vi "Topo & GridSpectr_DriftCorrection_v5.1- Cloud.vi"(6 "Internal use":string, 7 "Grid param":T2 {"height (m)" format="%#_6p"; "width (m)" format="%#_6p"; "center Y (m)" format="%#_6p"; "center X (m)" format="%#_6p"}, 8 "Error in (no error)":errorcluster, 9 "Points Y/Index Y":i32, 10 "Points X/Index X":i32, 11 "Method":enum16{"init", "run", "end"}(ring)=enum."end") -> (0 "Error out":errorcluster)   [LabVIEW 2014]
doc: "Example of a measurement VI to be used in the \"Experiments on a Grid\" tool as external VI.\n\nThis example measure the topography and spectroscopy data. The spectroscopy measurements are taken on a subgrid. The data are saved to a sxm and a binary file.\n\n- Nanonis Programming Interface -"
uses:
  <userlib>/Nanonis Prog Interface V5/Nanonis Prog Interface.lvlib
panel:
  in  "Drift Correction":bool
  in  "Set Session":bool
  in  "STS current step":dbl format="%#_6p"
  in  "tip Speed (m/s)":sgl=1e-08 format="%.2p"
  in  "Drift Correction 2":T1
  out "X drift":i32
  out "Y drift":i32
  in  "Channel index (0-23)":u8=14
  in  "File name":string="_3_mol_Chain_single_mol_KONDO"
  in  "STS Current":dbl=2e-10 format="%#_6p"
  in  "Imaging Current":dbl=8e-11 format="%#_6p"
  in  "zdrift \nDuration (s)":dbl
  in  "Correct z drift":bool
  out "Status":string="init"
  in  "Drift correction Pixels":i32=256 caption="Pixels for drift correction"
  out "Y Offset":dbl
  out "X Offset":dbl
  out "Points taken":dbl
  in  "Drift Correction every":i32=10
  in  "Y subgrid spacing":u16=1
  in  "X subgrid spacing":u16=1
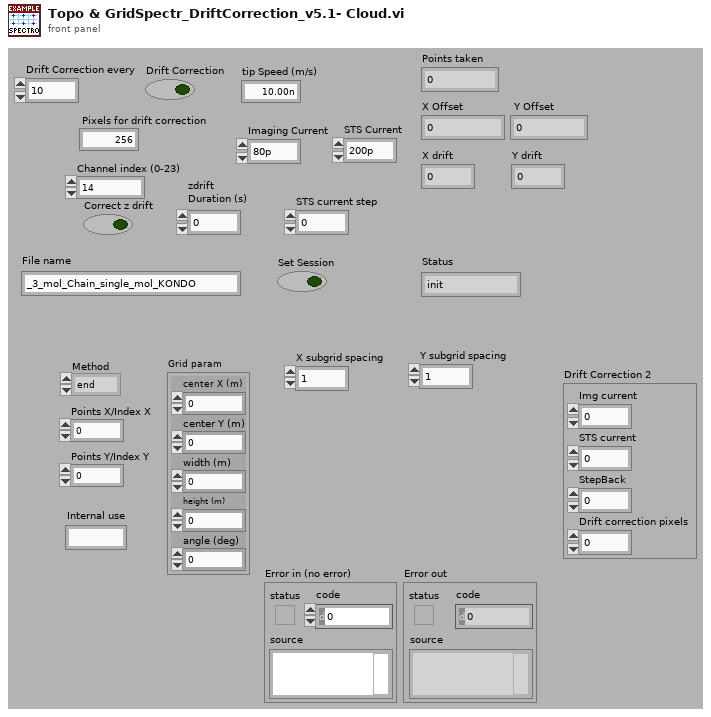
[diagram p1: front panel]
types:
  T1 = cluster{"Img current":dbl, "STS current":dbl, "StepBack":dbl, "Drift correction pixels":dbl}
  T2 = cluster{"center X (m)":sgl, "center Y (m)":sgl, "width (m)":sgl, "height (m)":sgl, "angle (deg)":sgl}
  T3 = enum16{"Header", "TOPO", "STS", "GRID", "GRIDCloud"}
  T4 = cluster{"center X":sgl, "center Y":sgl, "angle":sgl, "width":sgl, "height":sgl, "# pixels":i32, "# lines":i32}
  T5 = cluster{"Name":string, "Calibration":sgl, "Offset":sgl, "Channel index":i32}[]
  T6 = cluster{"up/down":bool, "time/line":sgl, "start time":timestamp, "end time":timestamp}
  T7 = cluster{"Z averaging time (s)":sgl, "Z offset (m)":sgl, "Initial settling time (s)":sgl}
  T8 = cluster{"Max. slew rate (V/s)":sgl, "Settling time (s)":sgl, "Integration time (s)":sgl}
  T9 = cluster{"End settling time (s)":sgl, "Z control time (s)":sgl}
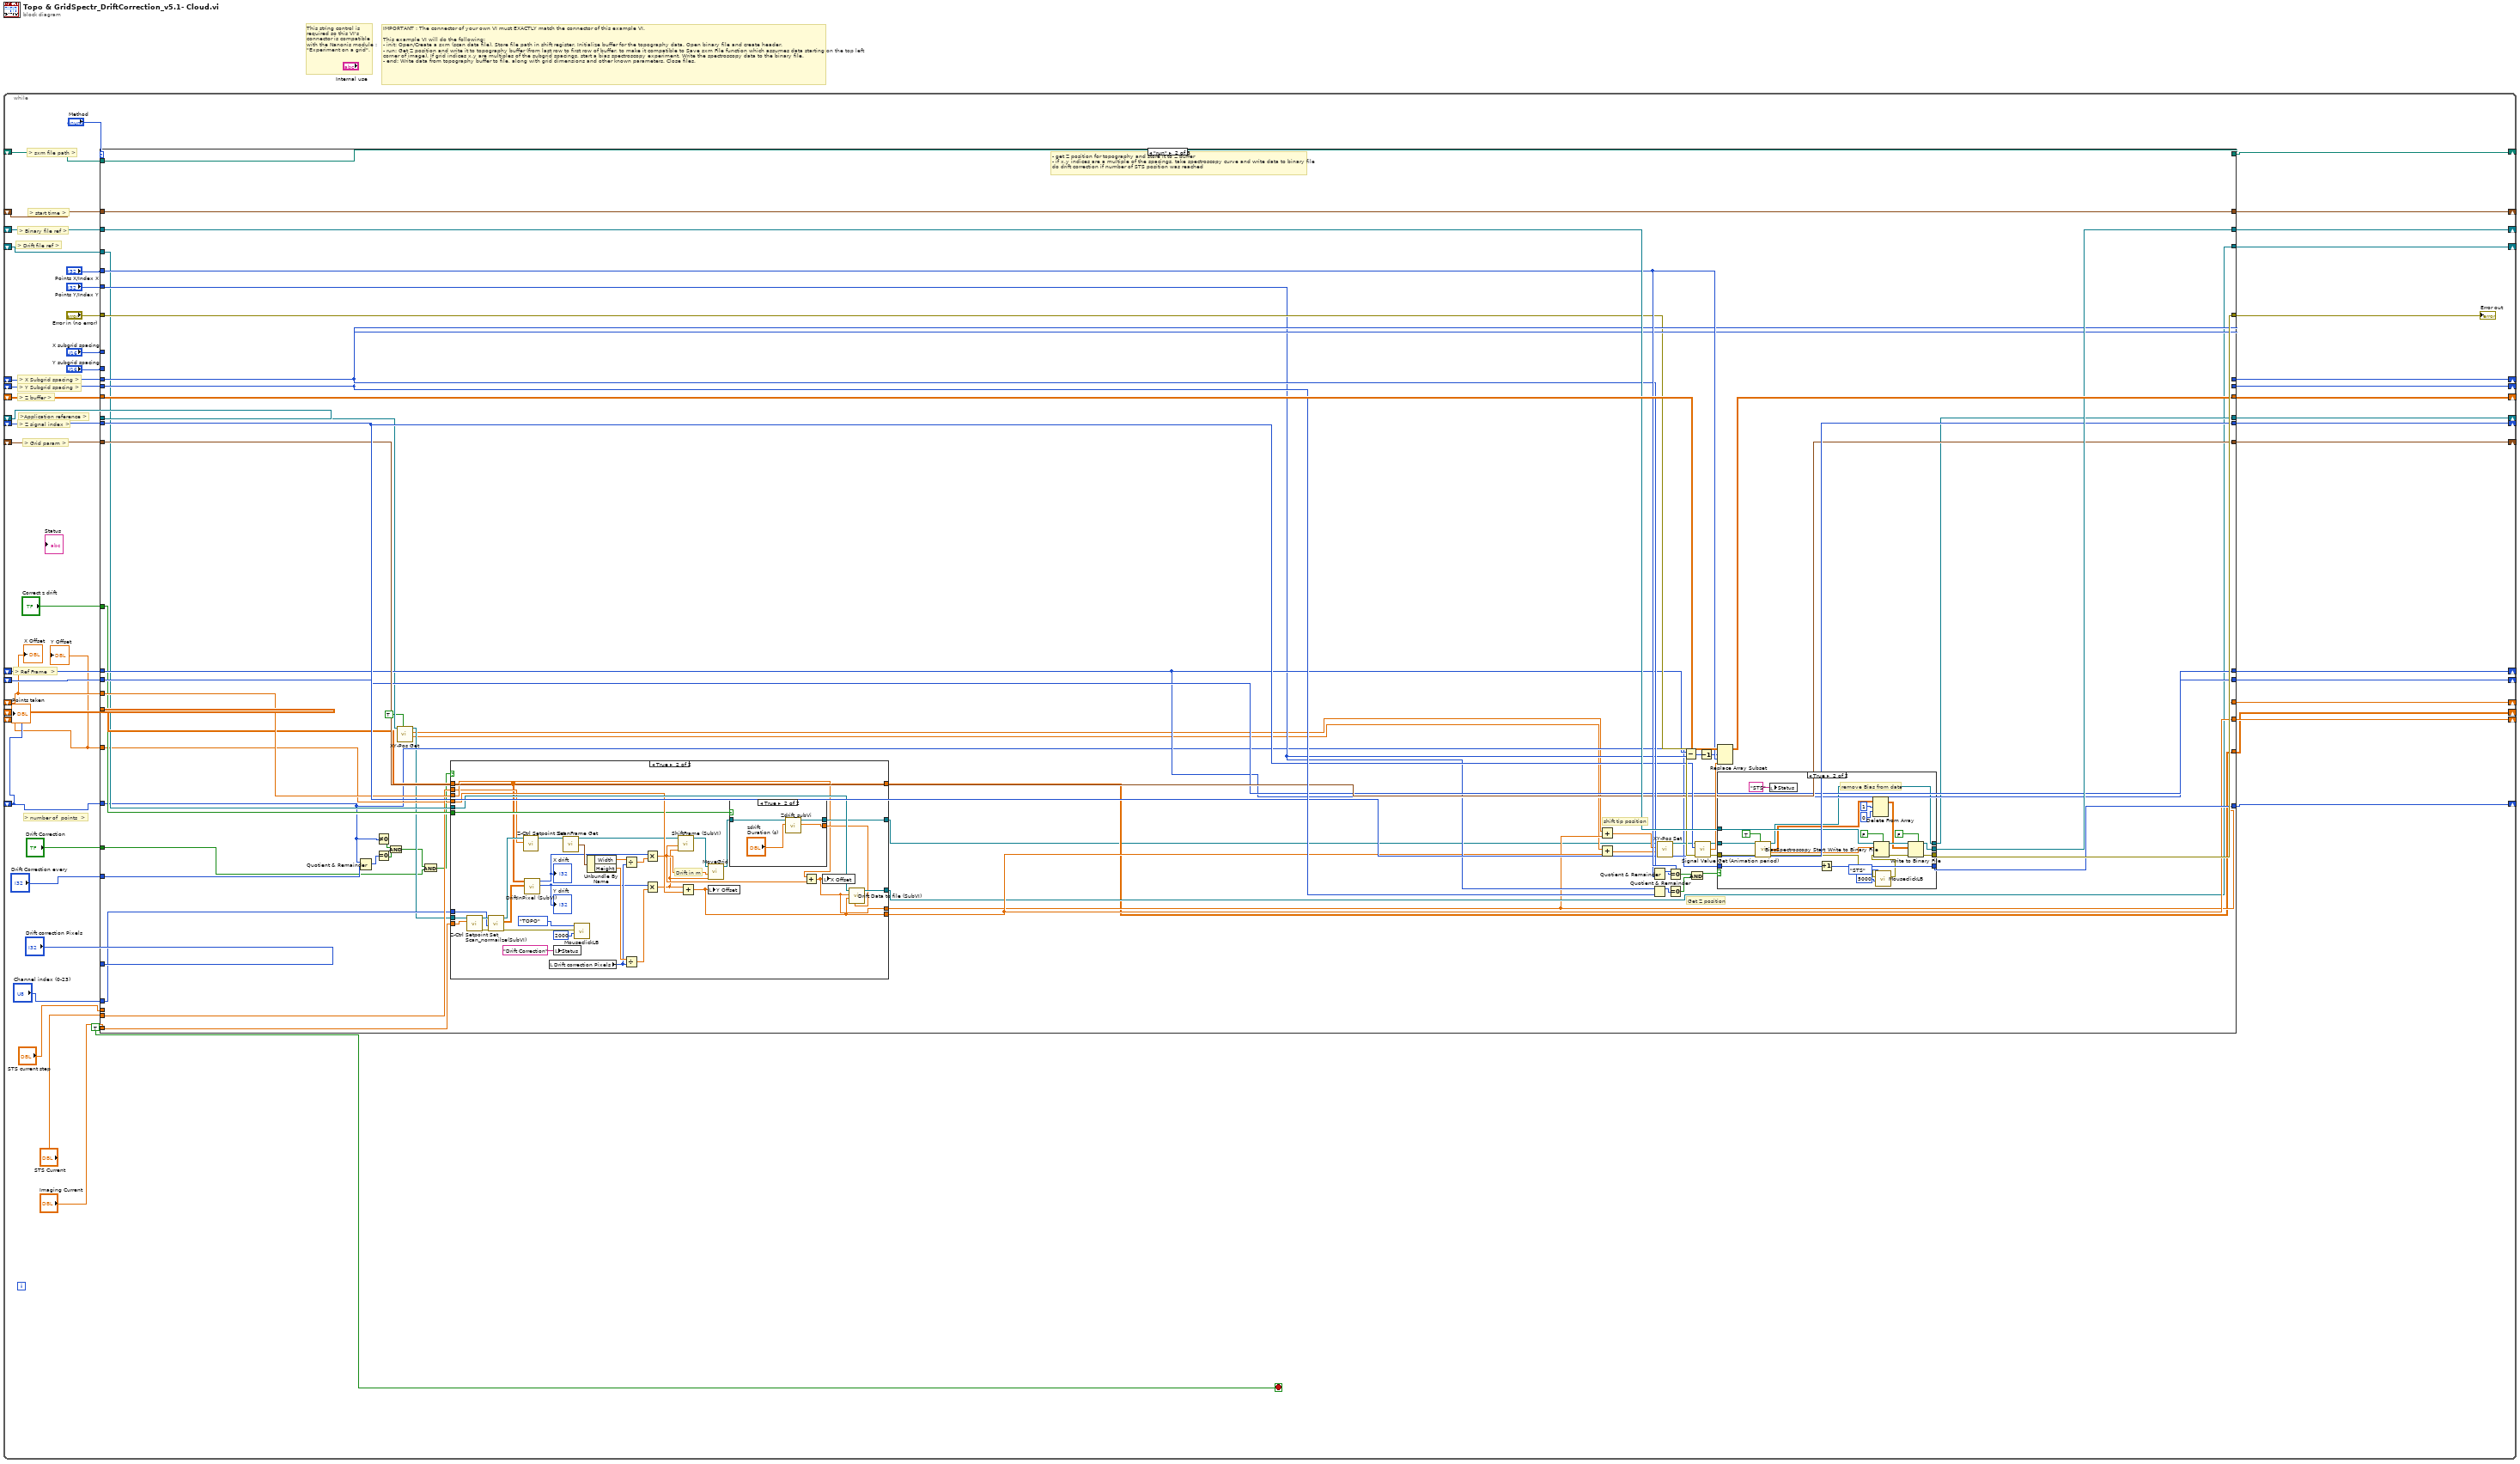
[diagram p0: block diagram]
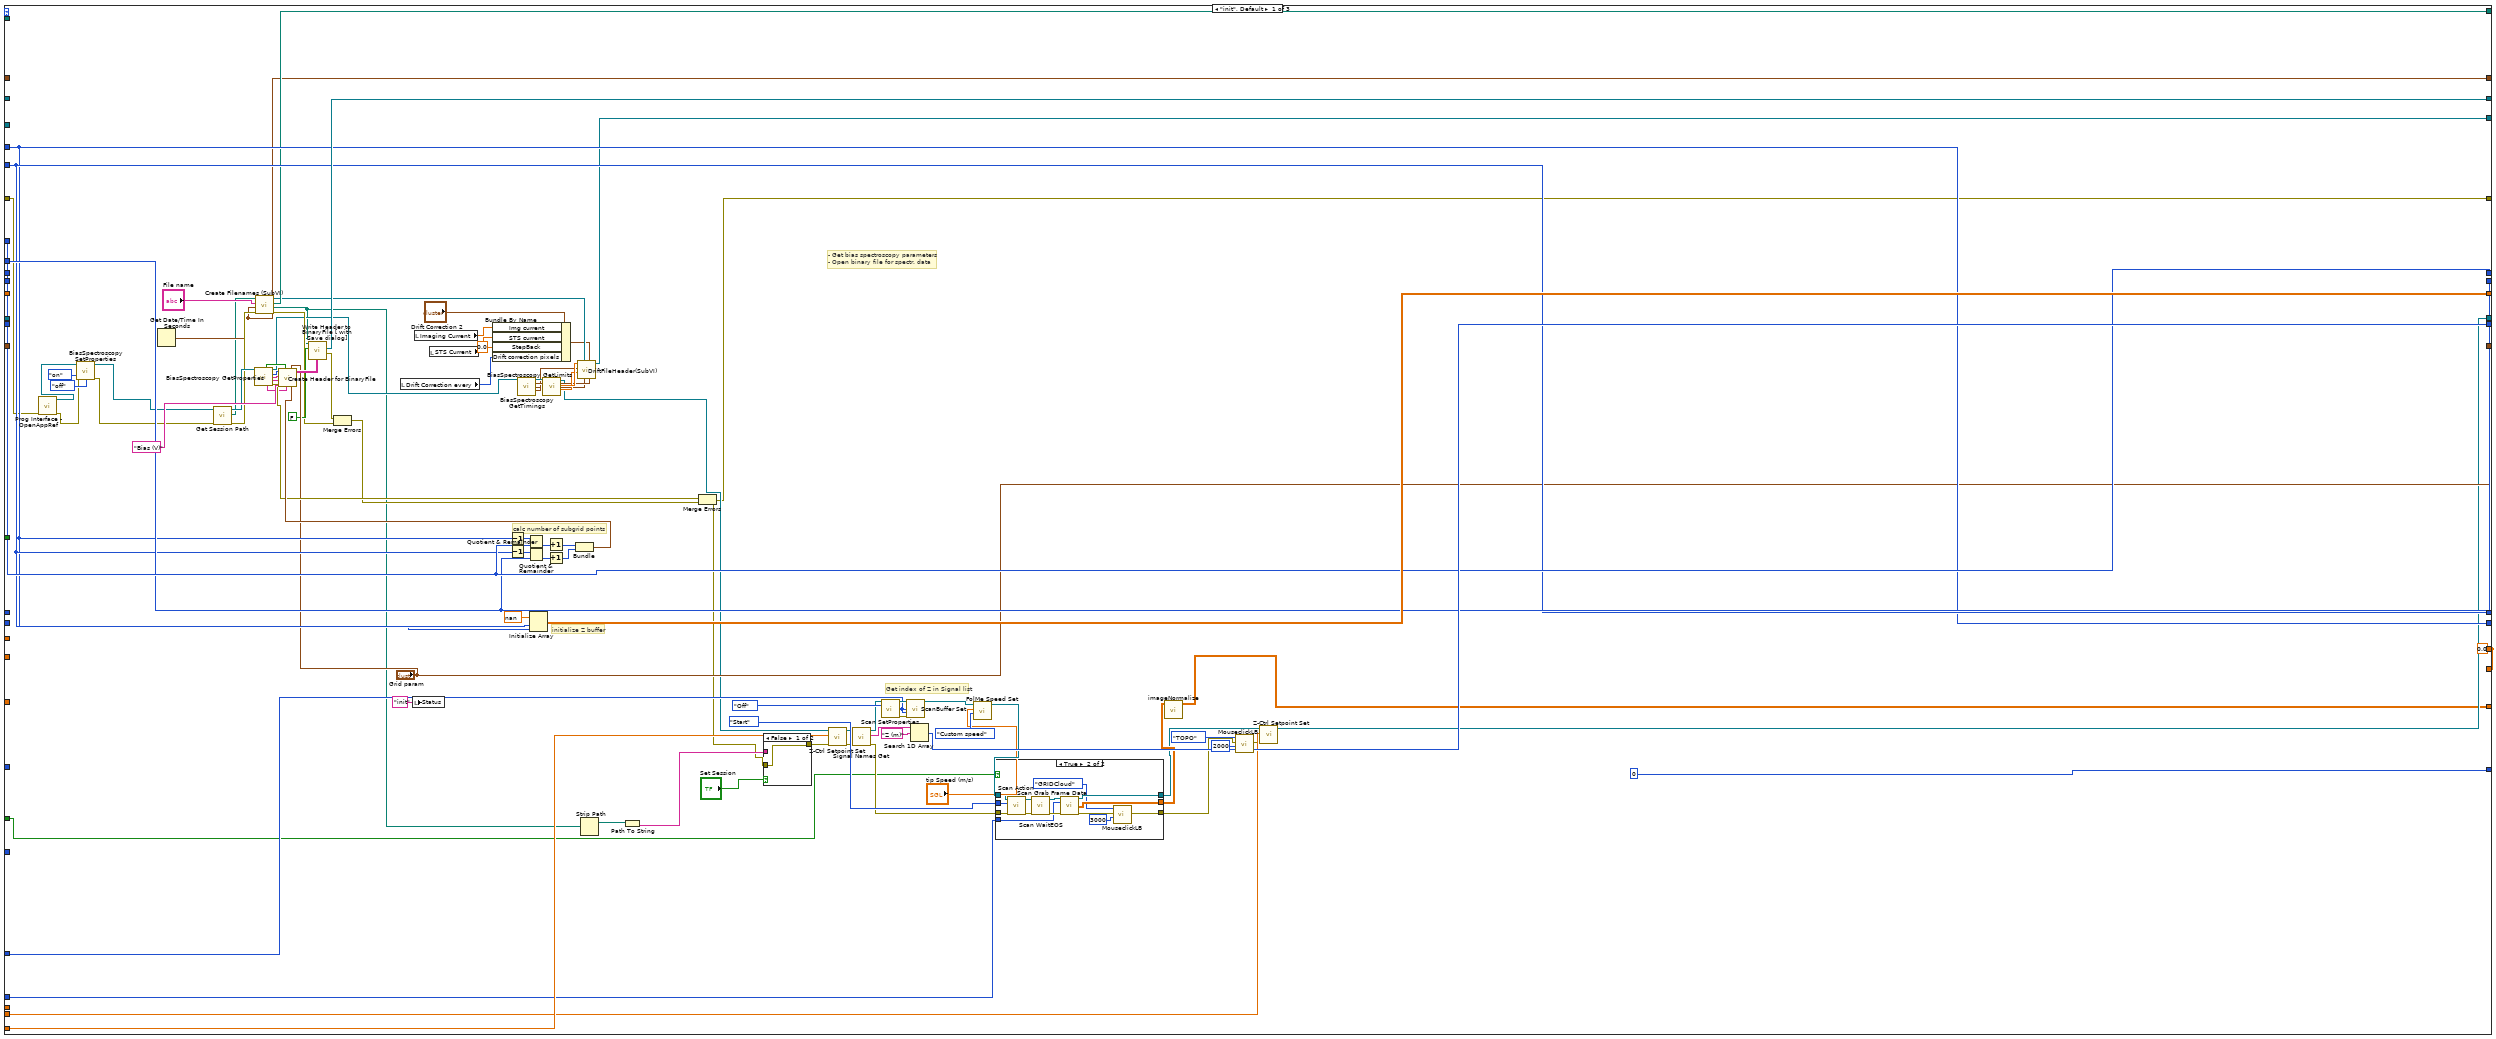
[diagram p2: hidden frame]
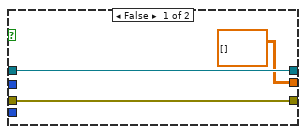
[diagram p3: hidden frame]
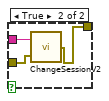
[diagram p4: hidden frame]
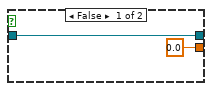
[diagram p6: hidden frame]
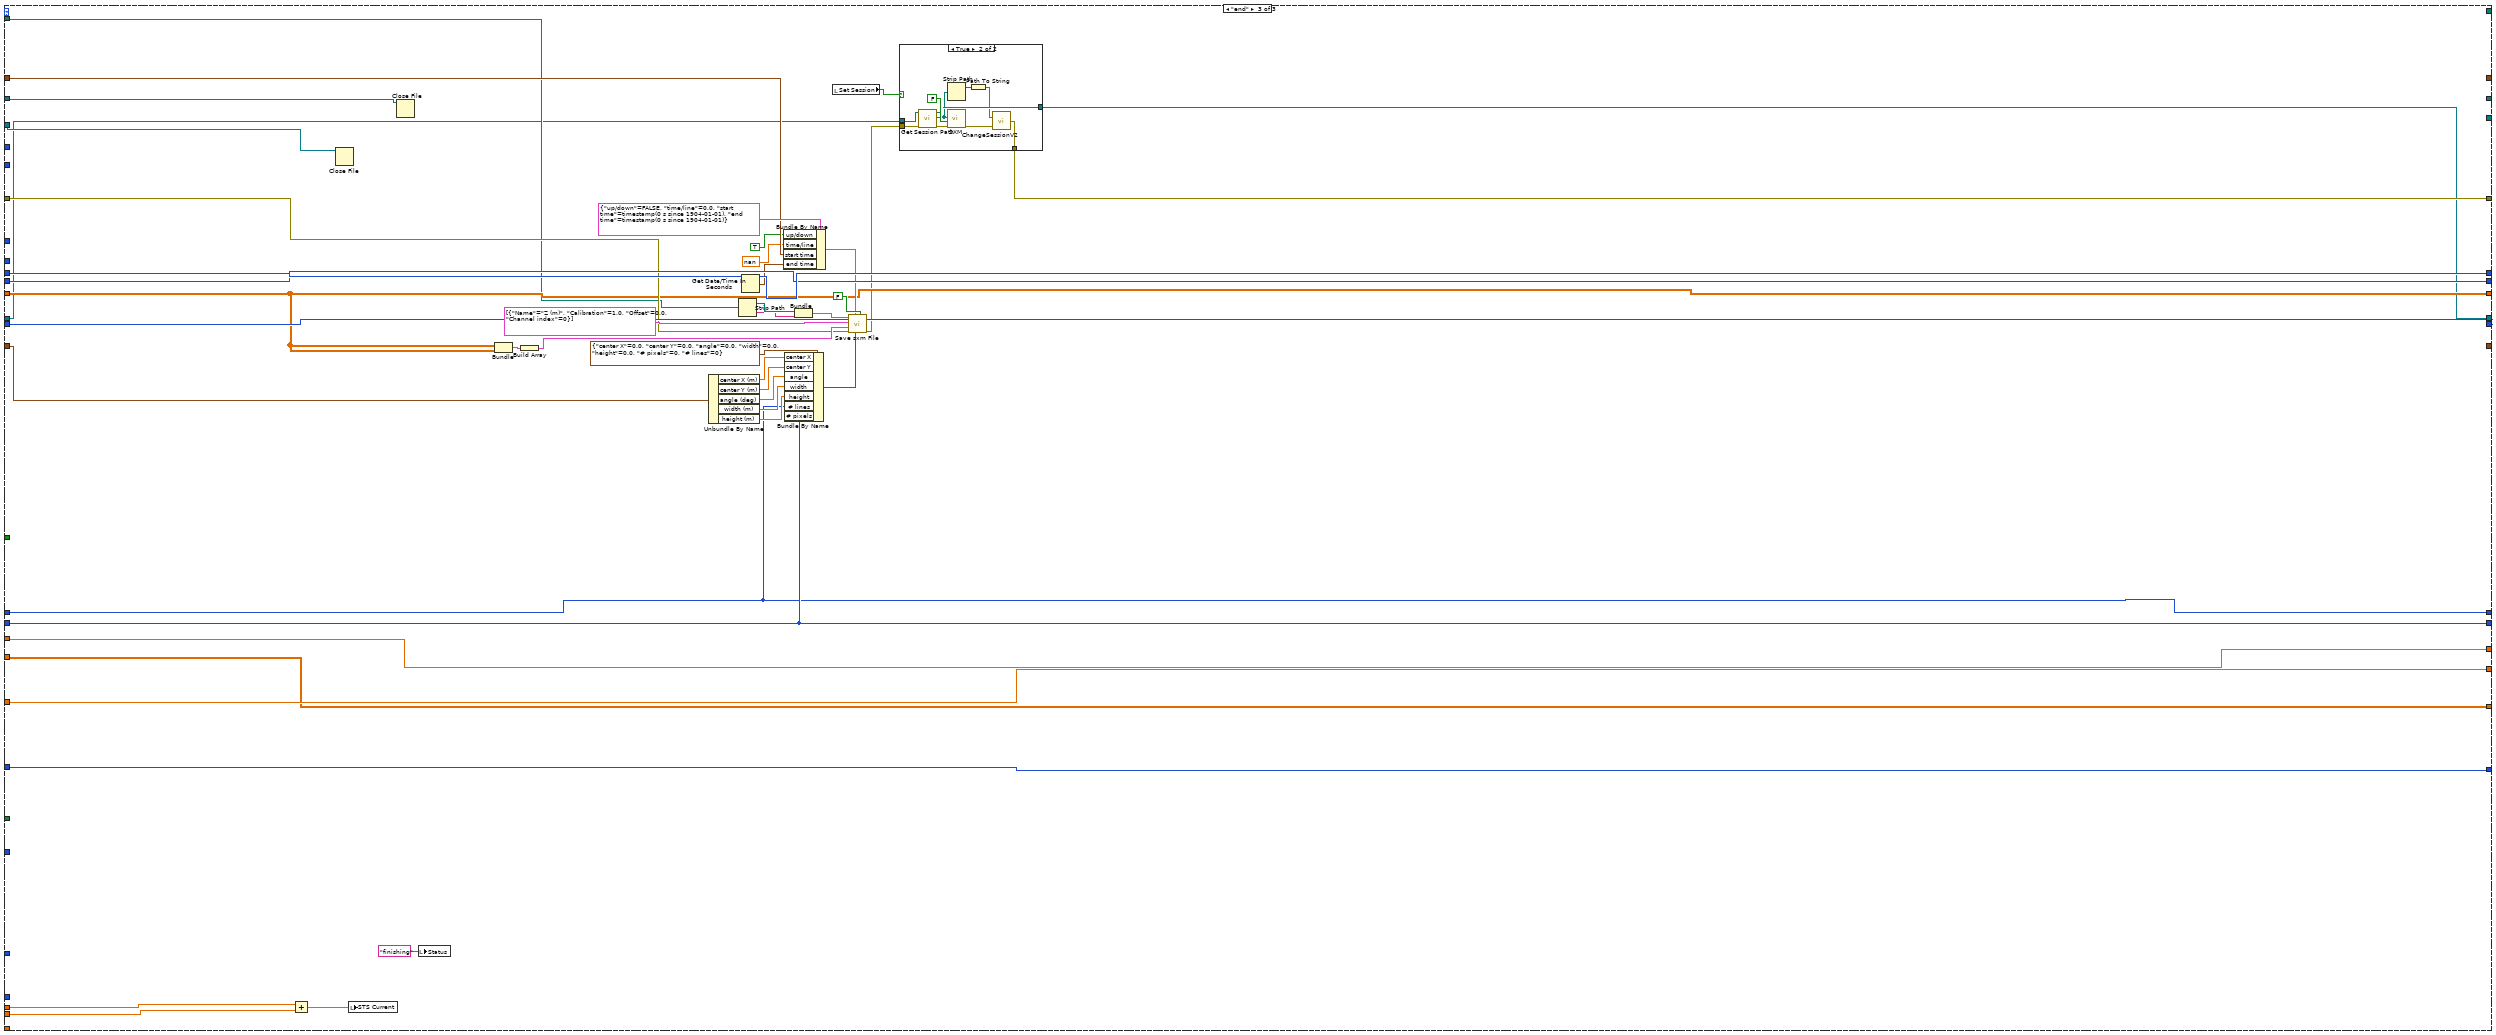
[diagram p8: hidden frame]
diagram:
  # "This string control is required so this VI's connector is compatible with the Nanonis module : \"Experiment on a grid\"."
  # "IMPORTANT : The connector of your own VI must EXACTLY match the connector of this example VI.\n\nThis example VI will do the following:\n- init: Open/Create a sxm (scan data file). Store file path in shift register. Initialize buffer for the topography data. Open binary file and create header.\n- run: Get Z position and write it to topography buffer (from last row to first row of buffer, to make it compatible to Save sxm File function which assumes data starting on the top left corner of image). If grid indices x,y are multiples of the subgrid spacings, start a bias spectroscopy experiment. Write the spectroscopy data to the binary file.\n- end: Write data from topography buffer to file, along with grid dimensions and other known parameters. Close files."
  n1 = while {
    shift-right: [w23] -> _
    shift-left: _ -> [w46]
    shift-right: [w41] -> _
    shift-left: _ -> [w40]
    shift-right: [w38] -> _
    shift-left: _ -> [w39]
    shift-right: [w37] -> _
    shift-left: _ -> [w36]
    shift-right: [w30] -> _
    shift-left: _ -> [w32]
    shift-right: [w31] -> _
    shift-left: _ -> [w33]
    shift-right: [w29] -> _
    shift-left: _ -> [w28]
    shift-right: [w27] -> _
    shift-left: _ -> [w26]
    shift-right: [w25] -> _
    shift-left: _ -> [w24]
    shift-right: [w22] -> _
    shift-left: _ -> [w21]
    shift-right: [w20] -> _
    shift-left: _ -> [w19]
    shift-right: [w18] -> _
    shift-left: _ -> [w11]
    shift-right: [w17] -> _
    shift-left: _ -> [w10]
    shift-right: [w16] -> _
    shift-left: _ -> [w13]
    shift-right: [w15] -> _
    shift-left: _ -> [w12]
    shift-right: [w8] -> _
    shift-left: _ -> [w7]
    stop <- TRUE stop-if-true
    # "> Drift file ref >"
    # "> number of  points  >"
    # "> Ref Frame  >"
    # "> Grid param >"
    # "> start time >"
    # ">Application reference >"
    # "> Y Subgrid spacing >"
    # "> X Subgrid spacing >"
    # "> Z signal index >"
    # "> Binary file ref >"
    # "> Z buffer >"
    # "> sxm file path >"
    n2 = case shown="\"run\"" "Method" {
      tunnel: [w97 w219 _] -> w23
      tunnel: w46 -> [_ w219 w300]
      tunnel: "Error in (no error)" -> [w64 w205 w323]
      tunnel: [w58 w218 w297] -> w44
      tunnel: "Points X/Index X" -> [w117 w213 _]
      tunnel: "Points Y/Index Y" -> [w118 w197 _]
      tunnel: [w141 w216 w312] -> w41
      tunnel: w40 -> [_ w217 w312]
      tunnel: w39 -> [_ w215 w301]
      tunnel: [w133 w214 _] -> w38
      tunnel: [w131 w203 w337] -> w37
      tunnel: w36 -> [_ w203 w337]
      tunnel: "X subgrid spacing" -> [w130 _ _]
      tunnel: "Y subgrid spacing" -> [w129 _ _]
      tunnel: w33 -> [_ w207 w336]
      tunnel: w32 -> [_ w206 w335]
      tunnel: [w130 w207 w336] -> w31
      tunnel: [w129 w206 w335] -> w30
      tunnel: [w76 w189 w295] -> w29
      tunnel: w28 -> [_ w171 w296]
      tunnel: ["Grid param" w200 _] -> w27
      tunnel: w26 -> [_ w200 w322]
      tunnel: [w96 w201 _] -> w25
      tunnel: w24 -> [_ w201 w330]
      tunnel: [w118 w198 w313] -> w22
      tunnel: w21 -> [_ w198 w313]
      tunnel: [w117 w199 w314] -> w20
      tunnel: w19 -> [_ w199 w314]
      tunnel: [w112 w179 w311] -> w18
      tunnel: [w112 w184 w309] -> w17
      tunnel: [w50 w176 w305] -> w16
      tunnel: [0 w194 w310] -> w15
      tunnel: w12 -> [_ w173 w310]
      tunnel: "Drift Correction every" -> [_ w192 _]
      tunnel: w13 -> [_ w183 w305]
      tunnel: w11 -> [_ w190 w311]
      tunnel: w10 -> [_ w174 w309]
      tunnel: "Drift correction Pixels" -> [w93 _ _]
      tunnel: [w91 w181 _] -> w8
      tunnel: w7 -> [_ w182 w306]
      tunnel: "Correct z drift" -> [_ w180 _]
      tunnel: "Imaging Current" -> [w103 w178 _]
      tunnel: "STS Current" -> [w100 w177 w302]
      tunnel: "Channel index (0-23)" -> [w94 w175 _]
      tunnel: "STS current step" -> [_ _ w304]
      tunnel: "Drift Correction" -> [w53 w163 _]
      frame "init", Default {
        w112 = 0.0
        # "- Get bias spectroscopy parameters\n- Open binary file for spectr. data"
        # "initialize Z buffer"
        # "calc number of subgrid points"
        # "Get index of Z in Signal list"
        n3 = call <userlib>:"Prog Interface - OpenAppRef.vi"("Error in (no error)"=w64) -> ("Error out"=w63:errorcluster, "Application reference"=w66:refnum<vi>)  [unwired: 5 in]
        n4 = call <userlib>:"BiasSpectroscopy SetProperties.vi"("Application ref in"=w66, "Autosave (no change)"=enum16{"no change", "on", "off"}."on", "Error in (no error)"=w63, "Save dialog"=enum16{"no change", "on", "off"}."off") -> ("Application ref out"=w65:refnum<vi>, "Error out"=w62:errorcluster)  [unwired: 10 in]
        n5 = Get Date/Time In Seconds() -> (seconds since 1Jan1904=w96:timestamp)
        n6 = call <userlib>:"Get Session Path.vi"("error in (no error)"=w62, "Application ref in"=w65) -> ("error out"=w98:errorcluster, "Session path"=w69:path, "Application ref out"=w99:refnum<vi>)  [unwired: 7 in]
        n7 = call <userlib>:"BiasSpectroscopy GetProperties.vi"("Application ref in"=w99) -> ("Backward sweep"=w137:bool, "Application ref out"=w75:refnum<vi>, "Number of points"=w120:i32, "Channels"=w119:string[], "Parameters"=w135:string[], "Fixed parameters"=w122:string[], "Error out"=w134:errorcluster)  [unwired: 6 in, 2 out]
        n8 = call "Create Filenames (SubVI).vi"("error in (no error)"=w98, "seconds since 1Jan1904"=w96, "File name"="File name", "Session path"=w69) -> ("error out"=w77:errorcluster, "binFilePath"=w59:path, "topoFilePath"=w97:path, "Drift File out"=w92:refnum<file>)  [unwired: 4 in]
        n9 = local read "Drift Correction every"() -> (w86:i32)
        n10 = local write "Status"("init" ("Status")) -> ()
        n11 = local read "Imaging Current"() -> (w88:dbl)
        n12 = local read "STS Current"() -> (w87:dbl)
        n13 = Bundle By Name(cluster="Drift Correction 2", "Img current"=w88, "STS current"=w87, "StepBack"=0.0, "Drift correction pixels"=w86) -> (w89:T1)
        n14 = Decrement(x=w117) -> (x-1=w128:i32)
        n15 = Decrement(x=w118) -> (x-1=w127:i32)
        n16 = call <userlib>:"BiasSpectroscopy GetTimings.vi"("Application ref in"=w75) -> ("Application ref out"=w85:refnum<vi>, "Initialization"=w82:T7, "Sweep Timing"=w80:T8, "End of Sweep"=w81:T9)  [unwired: 10 in, 1 out]
        n17 = Quotient & Remainder(x=w128, y=w130) -> (floor(x/y)=w126:i32)  [unwired: 1 out]
        n18 = Quotient & Remainder(x=w127, y=w129) -> (floor(x/y)=w125:i32)  [unwired: 1 out]
        n19 = Initialize Array(sgl nan ("element"), w118, w117) -> (w141:sgl[][])
        n20 = call <userlib>:"BiasSpectroscopy GetLimits.vi"("Application ref in"=w85) -> ("End value (V)"=w83:sgl, "Start value (V)"=w84:sgl, "Application ref out"=w74:refnum<vi>)  [unwired: 5 in, 1 out]
        n21 = Increment(x=w126) -> (x+1=w124:i32)
        n22 = Increment(x=w125) -> (x+1=w123:i32)
        n23 = Bundle(w124, w123) -> (w136:cluster{i32, i32})  [unwired: 1 in]
        n24 = call <userlib>:"Create Header for BinaryFile.vi"("Grid points"=w136, "Grid param"="Grid param", "Fixed parameters"=w122, "Backward sweep"=w137, "Sweep signal"="Bias (V)" ("Sweep Signal"), "Parameters"=w135, "Channels"=w119, "Points per sweep"=w120) -> ("Header (fixed attributes)"=w139:string[][])  [unwired: 3 in]
        n25 = call <userlib>:"Write Header to BinaryFile [ with Save dialog].vi"("Fixed Attributes"=w139, "Show Dialog? (T)"=FALSE, "Filename"=w59) -> ("Error out"=w78:errorcluster, "File ref"=w133:refnum<file>)  [unwired: 5 in, 2 out]
        n26 = Merge Errors(w78, w77) -> (w79:errorcluster)
        n27 = call "DriftFileHeader(SubVI).vi"("Initialization"=w82, "Drift Correction"=w89, "Sweep Timing"=w80, "Byte Stream File in"=w92, "End value (V)"=w83, "End of Sweep"=w81, "Start value (V)"=w84) -> ("Byte Stream File out"=w91:refnum<file>)  [unwired: 4 in]
        n28 = Strip Path(path=w59) -> (stripped path=w61:path)  [unwired: 1 out]
        n29 = Path To String(path=w61) -> (string=w60:string)
        n30 = Merge Errors(w134, w79) -> (w58:errorcluster)
        n31 = case shown="False" "Set Session" {
          tunnel: w60 -> [_ w162]
          tunnel: w58 -> [w159 w161]
          tunnel: [w159 w160] -> w57
          frame False {
          }
          frame True {
            n32 = call "ChangeSessionV2.vi"("error in (no error)"=w161, "Session"=w162) -> ("error out"=w160:errorcluster)
          }
        }
        n33 = call <userlib>:"Z-Ctrl Setpoint Set.vi"("error in (no error)"=w57, "Z Controller setpoint"=w103, "Application ref in"=w74) -> ("error out"=w102:errorcluster, "Application ref out"=w104:refnum<vi>)  [unwired: 7 in]
        n34 = call <userlib>:"Signal Names Get.vi"("error in (no error)"=w102, "Application ref in"=w104) -> ("error out"=w113:errorcluster, "Signals Names"=w121:string[], "Application ref out"=w108:refnum<vi>)  [unwired: 5 in]
        n35 = call <userlib>:"Scan SetProperties.vi"("Application ref in"=w108, "Continuous scan"=enum16{"No change", "On", "Off"}."Off") -> ("Application ref out"=w110:refnum<vi>, "Error out"=w109:errorcluster)  [unwired: 12 in]
        n36 = call <userlib>:"ScanBuffer Set.vi"("Application ref in"=w110, "Pixels"=w93, "Lines"=w93, "error in (no error)"=w109) -> ("Application ref out"=w73:refnum<vi>)  [unwired: 10 in, 1 out]
        n37 = Search 1D Array(1D array=w121, element="Z (m)") -> (index of element=w131:i32)  [unwired: 1 in]
        n38 = call <userlib>:"FolMe Speed Set.vi"("Speed Setting (Custom)"=enum32{"Scan speed", "Custom speed"}."Custom speed", "Speed (m/s)"="tip Speed (m/s)", "Application ref in"=w73) -> ("Application ref out"=w72:refnum<vi>)  [unwired: 5 in, 1 out]
        n39 = case shown="True" w53 {
          tunnel: enum16{"Start", "Stop", "Pause", "Resume"}."Start" ("Scan action (Start)") -> [_ w154]
          tunnel: w113 -> [w144 w153]
          tunnel: [sgl[][] [] ("Scan frame data") w152] -> w105
          tunnel: [w143 w151] -> w101
          tunnel: w94 -> [_ w150]
          tunnel: w72 -> [w143 w149]
          tunnel: [w144 w147] -> w55
          frame False {
          }
          frame True {
            n40 = call <userlib>:"Scan Action.vi"("error in (no error)"=w153, "Scan action (Start)"=w154, "Application ref in"=w149) -> ("error out"=w158:errorcluster, "Application ref out"=w157:refnum<vi>)  [unwired: 6 in]
            n41 = call <userlib>:"Scan WaitEOS.vi"("error in (no error)"=w158, "Application ref in"=w157) -> ("error out"=w155:errorcluster, "Application ref out"=w156:refnum<vi>)  [unwired: 5 in, 2 out]
            n42 = call <userlib>:"Scan Grab Frame Data.vi"("Application ref in"=w156, "Channel index (0-23)"=w150, "error in (no error)"=w155) -> ("Application ref out"=w151:refnum<vi>, "Scan frame data"=w152:sgl[][], "error out"=w148:errorcluster)  [unwired: 8 in, 2 out]
            n43 = call "MouseclickLB.vi"("nMilliseconds"=3000, "error in (no error)"=w148, "Click"=T3."GRIDCloud") -> ("error out"=w147:errorcluster)  [unwired: 8 in]
          }
        }
        n44 = call "imageNormalize.vi"("Data"=w105) -> ("Array"=w50:dbl[][])  [unwired: 10 in]
        n45 = call "MouseclickLB.vi"("nMilliseconds"=2000, "error in (no error)"=w55, "Click"=T3."TOPO") -> ("error out"=w56:errorcluster)  [unwired: 8 in]
        n46 = call <userlib>:"Z-Ctrl Setpoint Set.vi"("error in (no error)"=w56, "Z Controller setpoint"=w100, "Application ref in"=w101) -> ("Application ref out"=w76:refnum<vi>)  [unwired: 7 in, 1 out]
      }
      frame "run" {
        # "shift tip position"
        # "Get Z position"
        # "- get Z position for topography and store it to Z buffer\n- if x,y indices are a multiple of the spacings, take spectroscopy curve and write data to binary file\ndo drift correction if number of STS position was reached"
        n47 = Quotient & Remainder(x=w173, y=w192) -> (x-y*floor(x/y)=w193:i32)  [unwired: 1 out]
        n48 = Not Equal To 0?(x=w173) -> (x != 0?=w172:bool)
        n49 = Equal To 0?(x=w193) -> (x = 0?=w191:bool)
        n50 = And(x=w172, y=w191) -> (x .and. y?=w165:bool)
        n51 = call <userlib>:"XY-Pos Get.vi"("Wait for newest data (F=False)"=TRUE, "Application ref in"=w171) -> ("Y (m)"=w167:sgl, "X (m)"=w168:sgl, "Application ref out"=w170:refnum<vi>)  [unwired: 5 in, 1 out]
        n52 = And(x=w165, y=w163) -> (x .and. y?=w164:bool)
        n53 = case shown="True" w164 {
          tunnel: w170 -> [w224 w245]
          tunnel: [w224 w251] -> w166
          tunnel: w183 -> [w221 w225]
          tunnel: [w223 w247] -> w179
          tunnel: [w222 w246] -> w184
          tunnel: w190 -> [w223 w249]
          tunnel: w174 -> [w222 w250]
          tunnel: [w221 w225] -> w176
          tunnel: w182 -> [w220 w254]
          tunnel: [w220 w253] -> w181
          tunnel: w180 -> [_ w248]
          tunnel: w178 -> [_ w244]
          tunnel: w177 -> [_ w242]
          tunnel: w175 -> [_ w237]
          frame False {
          }
          frame True {
            # "Drift in m"
            n54 = call <userlib>:"Z-Ctrl Setpoint Set.vi"("Z Controller setpoint"=w244, "Application ref in"=w245) -> ("error out"=w229:errorcluster, "Application ref out"=w241:refnum<vi>)  [unwired: 8 in]
            n55 = call "Scan_normailze(SubVI).vi"("error in (no error)"=w229, "Channel index (0-23)"=w237, "Application in"=w241) -> ("error out"=w228:errorcluster, "Array"=w234:dbl[][], "Application out"=w243:refnum<vi>)  [unwired: 6 in]
            n56 = call <userlib>:"Z-Ctrl Setpoint Set.vi"("Z Controller setpoint"=w242, "Application ref in"=w243) -> ("Application ref out"=w239:refnum<vi>)  [unwired: 8 in, 1 out]
            n57 = call "DriftInPixel (SubVI).vi"("New image"=w234, "Ref image"=w225) -> ("Y drift"=w235:i32, "X drift"=w236:i32)  [unwired: 7 in, 1 out]
            "Y drift" <- w235
            "X drift" <- w236
            n58 = local read "Drift correction Pixels"() -> (w238:i32)
            n59 = local write "Status"("Drift Correction" ("Status")) -> ()
            n60 = call <userlib>:"ScanFrame Get.vi"("Application ref in"=w239) -> ("Application ref out"=w240:refnum<vi>, "Size (m)"=w259:cluster{"Width":sgl, "Height":sgl})  [unwired: 10 in, 3 out]
            n61 = call "MouseclickLB.vi"("nMilliseconds"=2000, "error in (no error)"=w228, "Click"=enum16{"Header", "TOPO", "STS", "GRID"}."TOPO") -> ()  [unwired: 8 in, 1 out]
            n62 = Unbundle By Name(w259) -> ("Width"=w258:sgl, "Height"=w260:sgl)
            n63 = Divide(x=w258, y=w238) -> (x/y=w257:sgl)
            n64 = Divide(x=w260, y=w238) -> (x/y=w256:sgl)
            n65 = Multiply(x=w236, y=w257) -> (x*y=w231:sgl)
            n66 = Multiply(x=w235, y=w256) -> (x*y=w230:sgl)
            n67 = call "ShiftFrame (SubVI).vi"("Y shift"=w230, "X shift"=w231, "Application in"=w240) -> ("Application out"=w233:refnum<vi>)  [unwired: 8 in]
            n68 = Add(x=w230, y=w250) -> (x+y=w246:dbl)
            n69 = call "MoveGrid.vi"("y"=w230, "x"=w231, "Application ref in"=w233) -> ("Application ref out"=w232:refnum<vi>)  [unwired: 7 in, 1 out]
            n70 = local write "Y Offset"(w246) -> ()
            n71 = case shown="True" w248 {
              tunnel: [0.0 ("z drift") w266] -> w252
              tunnel: w232 -> [w261 w265]
              tunnel: [w261 w264] -> w251
              frame False {
              }
              frame True {
                n72 = call "Zdrift_subVi.vi"("Duration"="zdrift \nDuration (s)", "Application in"=w265) -> ("z drift"=w266:dbl, "Application out"=w264:refnum<vi>)  [unwired: 7 in, 1 out]
              }
            }
            n73 = Add(x=w249, y=w231) -> (x+y=w247:dbl)
            n74 = local write "X Offset"(w247) -> ()
            n75 = call "Drift Data to file (SubVI).vi"("z drift"=w252, "y Drift"=w246, "X drift"=w247, "Byte Stream File in"=w254) -> ("Byte Stream File out"=w253:refnum<file>)  [unwired: 7 in]
          }
        }
        n76 = Add(x=w168, y=w179) -> (x+y=w186:dbl)
        n77 = Add(x=w167, y=w184) -> (x+y=w185:dbl)
        n78 = Quotient & Remainder(x=w213, y=w207) -> (x-y*floor(x/y)=w212:i32)  [unwired: 1 out]
        n79 = Quotient & Remainder(x=w197, y=w206) -> (x-y*floor(x/y)=w211:i32)  [unwired: 1 out]
        n80 = call <userlib>:"XY-Pos Set.vi"("Y (m)"=w185, "X (m)"=w186, "Application ref in"=w166) -> ("Application ref out"=w187:refnum<vi>)  [unwired: 5 in, 1 out]
        n81 = Equal To 0?(x=w212) -> (x = 0?=w210:bool)
        n82 = Equal To 0?(x=w211) -> (x = 0?=w209:bool)
        n83 = Subtract(x=w198, y=w197) -> (x-y=w196:i32)
        n84 = And(x=w210, y=w209) -> (x .and. y?=w208:bool)
        n85 = call <userlib>:"Signal Value Get (Animation period).vi"("error in (no error)"=w205, "Signal index (0-47)"=w203, "Application ref in"=w187) -> ("error out"=w204:errorcluster, "Signal value"=w202:sgl, "Application ref out"=w188:refnum<vi>)  [unwired: 5 in]
        n86 = Decrement(x=w196) -> (x-1=w195:i32)
        n87 = Replace Array Subset(array=w217, new element=w202, index (row)=w195, index (col)=w213) -> (w216:sgl[][])
        n88 = case shown="True" w208 {
          tunnel: [w269 w278] -> w218
          tunnel: w215 -> [w270 w293]
          tunnel: [w270 w291] -> w214
          tunnel: w204 -> [w269 w290]
          tunnel: w188 -> [w268 w282]
          tunnel: [w268 w281] -> w189
          tunnel: [w267 w276] -> w194
          tunnel: w173 -> [w267 w277]
          frame False {
            # "Point indices aren't multiple of subgrid spacing\n=> no spectroscopy at this point"
          }
          frame True {
            # "remove Bias from data"
            n89 = call <userlib>:"BiasSpectroscopy Start.vi"("Application ref in"=w282, "Get data (F)"=TRUE ("Get Data (F)"), "Error in (no error)"=w290) -> ("Application ref out"=w281:refnum<vi>, "Data"=w289:sgl[][], "Parameters"=w288:sgl[], "Error out"=w273:errorcluster)  [unwired: 8 in, 1 out]
            n90 = local write "Status"("STS" ("Status")) -> ()
            n91 = Increment(x=w277) -> (x+1=w276:i32)
            n92 = Delete From Array(array=w289, length=1, index (row)=0 ("index")) -> (array with subset deleted=w287:sgl[][])  [unwired: 1 in, 1 out]
            n93 = call "MouseclickLB.vi"("nMilliseconds"=5000, "error in (no error)"=w273, "Click"=enum16{"Header", "TOPO", "STS", "GRID"}."STS") -> ("error out"=w274:errorcluster)  [unwired: 8 in]
            n94 = Write to Binary File(file (use dialog)=w293, data=w288, error in=w274, 5:FALSE ("prepend array or string size? (T)")) -> (refnum out=w292:refnum<file>, error out=w279:errorcluster)  [unwired: 2 in, 1 out]
            n95 = Write to Binary File(file (use dialog)=w292, data=w287, error in=w279, 5:FALSE ("prepend array or string size? (T)")) -> (refnum out=w291:refnum<file>, error out=w278:errorcluster)  [unwired: 2 in, 1 out]
          }
        }
      }
      frame "end" {
        n96 = Add(x=w304, y=w302) -> (x+y=w303:dbl)
        n97 = Close File(refnum=w306) -> ()  [unwired: 1 in, 2 out]
        n98 = local write "STS Current"(w303) -> ()
        n99 = Close File(refnum=w301) -> ()  [unwired: 1 in, 2 out]
        n100 = local write "Status"("finishing" ("Status")) -> ()
        n101 = Bundle(w312, w312) -> (w334:cluster{sgl[][], sgl[][]})  [unwired: 1 in]
        n102 = Build Array(w334) -> (w333:cluster{sgl[][], sgl[][]}[])
        n103 = Unbundle By Name(w322) -> ("center X (m)"=w320:sgl, "center Y (m)"=w319:sgl, "angle (deg)"=w318:sgl, "width (m)"=w317:sgl, "height (m)"=w316:sgl)
        n104 = Strip Path(path=w300) -> (stripped path=w326:path, name=w325:string)
        n105 = Get Date/Time In Seconds() -> (seconds since 1Jan1904=w308:timestamp)
        n106 = Bundle By Name(cluster=T6 {"up/down"=FALSE, "time/line"=0.0, "start time"=timestamp(0 s since 1904-01-01), "end time"=timestamp(0 s since 1904-01-01)} ("Scan param"), "up/down"=TRUE, "time/line"=sgl nan ("input 7"), "start time"=w330, "end time"=w308) -> (w329:T6)
        n107 = Bundle By Name(cluster=T4 {"center X"=0.0, "center Y"=0.0, "angle"=0.0, "width"=0.0, "height"=0.0, "# pixels"=0, "# lines"=0} ("Scanfield"), "center X"=w320, "center Y"=w319, "angle"=w318, "width"=w317, "height"=w316, "# lines"=w313, "# pixels"=w314) -> (w315:T4)
        n108 = Bundle("stripped path"=w326, "name"=w325) -> (w324:cluster{"stripped path":path, "name":string})  [unwired: 1 in]
        n109 = local read "Set Session"() -> (w294:bool)
        n110 = call <userlib>:"Save sxm File.vi"("Auto file naming? (T)"=FALSE, "Scanfield"=w315, "Scan param"=w329, "error in (no error)"=w323, "Channels data"=w333, "Channels config"=T5 [{"Name"="Z (m)", "Calibration"=1.0, "Offset"=0.0, "Channel index"=0}], "Filename control"=w324) -> ("error out"=w298:errorcluster)  [unwired: 2 in, 2 out]
        n111 = case shown="True" w294 {
          tunnel: w298 -> [w338 w347]
          tunnel: [w338 w346] -> w297
          tunnel: w296 -> [w339 w344]
          tunnel: [w339 w343] -> w295
          frame False {
          }
          frame True {
            n112 = call <userlib>:"Get Session Path.vi"("error in (no error)"=w347, "Application ref in"=w344) -> ("error out"=w349:errorcluster, "Session path"=w342:path, "Application ref out"=w343:refnum<vi>)  [unwired: 7 in]
            n113 = Strip Path(path=w342) -> (stripped path=w341:path)  [unwired: 1 out]
            n114 = call "SXM.vi"("Path"=w342, "Delete"=FALSE, "error in"=w349) -> ("error out"=w348:errorcluster)  [unwired: 7 in]
            n115 = Path To String(path=w341) -> (string=w340:string)
            n116 = call "ChangeSessionV2.vi"("error in (no error)"=w348, "Session"=w340) -> ("error out"=w346:errorcluster)
          }
        }
      }
    }
    "Error out" <- w44
    "Points taken" <- w12
    "X Offset" <- w11
    "Y Offset" <- w10
  }
